vi "run.start.vi"(8 "error in":errorcluster, 11 "Run in":refnum<class "Run.lvclass">) -> (0 "error out":errorcluster, 3 "Run out":refnum<class "Run.lvclass">)   [LabVIEW 2020, in "Run.lvclass"]
doc: "Returns the run's start time."
uses:
  Run.lvclass
  Run.lvclass/Run.ctl
  client.lvlib
panel:
  out "out_millis out":dbl
  in  "out_millis":dbl
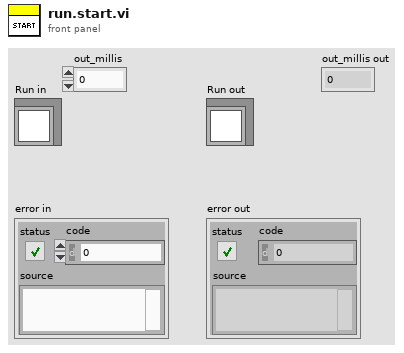
[diagram p1: front panel]
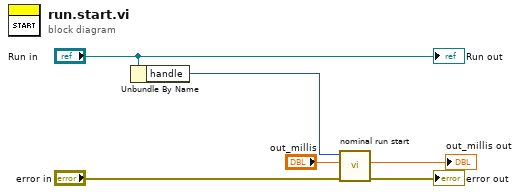
[diagram p0: block diagram]
diagram:
  n1 = Unbundle By Name("Run in") -> ("handle"=w4:i32)
  n2 = call "nominal run start.vi"("error in (no error)"="error in", "out_millis"="out_millis", "run"=w4) -> ("error out"=→"error out":errorcluster, "out_millis out"=→"out_millis out":dbl)  [unwired: 6 in, 1 out]
  "Run out" <- "Run in"
